vi "Get All Classes.vi"(8 "error in (no error)":errorcluster) -> (0 "error out":errorcluster, 3 "VI Server Classes[]":T1(array[cluster]))   [LabVIEW 2023]
doc: "<b> </b> <b> </b>\n© 2017 Q Software Innovations, LLC\nwritten by Quentin \"Q\" Alldredge\nproduced in LabVIEW 2015\n\nsupport@qsoftwareinnovations.com\nwww.qsoftwareinnovations.com\n\nAll rights reserved.\n\nRedistribution and use in source and binary forms, with or without modification, are permitted provided that the following conditions are met:\n\n * Redistributions of source code must retain the above copyright notice, this list of conditions and the following disclaimer.\n * Redistributions in binary form must reproduce the above copyright notice, this list of conditions and the following disclaimer in the documentation and/or other materials provided with the distribution.\n * Neither the name of Q Software Innovations, LLC. nor the names of its contributors may be used to endorse or promote products derived from this software without specific prior written permission.\n\nTHIS SOFTWARE IS PROVIDED BY THE COPYRIGHT HOLDERS AND CONTRIBUTORS \"AS IS\" AND ANY EXPRESS OR IMPLIED WARRANTIES, INCLUDING, BUT NOT LIMITED TO, THE IMPLIED WARRANTIES OF MERCHANTABILITY AND FITNESS FOR A PARTICULAR PURPOSE ARE DISCLAIMED. IN NO EVENT SHALL THE COPYRIGHT OWNER OR CONTRIBUTORS BE LIABLE FOR ANY DIRECT, INDIRECT, INCIDENTAL, SPECIAL, EXEMPLARY, OR CONSEQUENTIAL DAMAGES (INCLUDING, BUT NOT LIMITED TO, PROCUREMENT OF SUBSTITUTE GOODS OR SERVICES; LOSS OF USE, DATA, OR PROFITS; OR BUSINESS INTERRUPTION) HOWEVER CAUSED AND ON ANY THEORY OF LIABILITY, WHETHER IN CONTRACT, STRICT LIABILITY, OR TORT (INCLUDING NEGLIGENCE OR OTHERWISE) ARISING IN ANY WAY OUT OF THE USE OF THIS SOFTWARE, EVEN IF ADVISED OF THE POSSIBILITY OF SUCH DAMAGE."
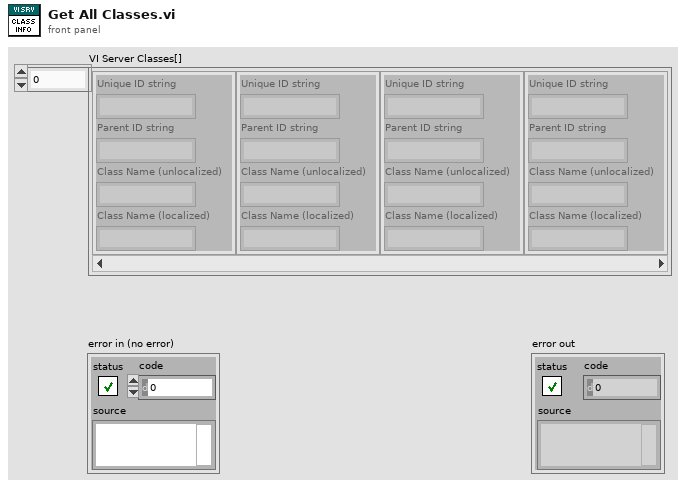
[diagram p1: front panel]
types:
  T1 = cluster{"Unique ID string":string, "Parent ID string":string, "Class Name (unlocalized)":string, "Class Name (localized)":string}[]
  T2 = typedef "ASC_ArrayOfUniqueIDStringParentIDStringName.ctl" = T3[]
  T3 = typedef "ASC_UniqueIDStringParentIDStringName.ctl" = cluster{"Unique ID string":string, "Parent ID string":string, "Class Name (unlocalized)":string, "Class Name (localized)":string}
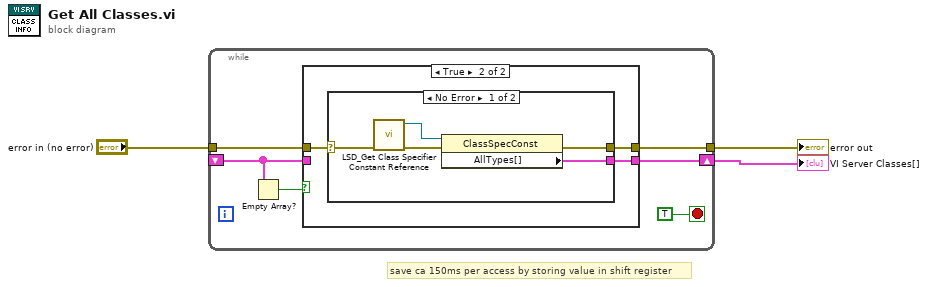
[diagram p0: block diagram]
diagram:
  # "save ca 150ms per access by storing value in shift register"
  n1 = while {
    shift-right: [w7] -> w3
    shift-left: _ -> [w6]
    tunnel: "error in (no error)" -> [w9]
    tunnel: [w8] -> w1
    stop <- TRUE stop-if-true
    n2 = Empty Array?(array=w6) -> (empty?=w4:bool)
    n3 = case shown="True" w4 {
      tunnel: w9 -> [w10 w14]
      tunnel: [w10 w13] -> w8
      tunnel: [w11 w12] -> w7
      tunnel: w6 -> [w11 _]
      frame False {
      }
      frame True {
        n4 = case shown="No Error" w14 {
          selector: w14 -> [w19 w20]
          tunnel: [w17 w20] -> w13
          tunnel: [w15 _] -> w12
          frame No Error {
            n5 = call <resource>:"LSD_Get Class Specifier Constant Reference.vi"("error in (no error)"=w19) -> ("error out"=w18:errorcluster, "specific class reference"=w16:refnum<vi>)  [unwired: 9 in]
            n6 = property class="ClassSpecConst"(reference=w16, error in=w18) -> (error out=w17:errorcluster, "AllTypes[]"=w15:T2)  [unwired: 1 out]
          }
          frame Error {
          }
        }
      }
    }
  }
  "error out" <- w1
  "VI Server Classes[]" <- w3
